vi "grSim Robot Command.vi"(9 "Array In":u8[](array[numeric]), 11 "Robots":T1) -> (1 "Array":u8[](array[numeric]))   [LabVIEW 2018]
uses:
  Convert AI Robot to Robot Command Folder/grSim/grSim Robot Command.ctl
  Varint Encoder uint32.vi
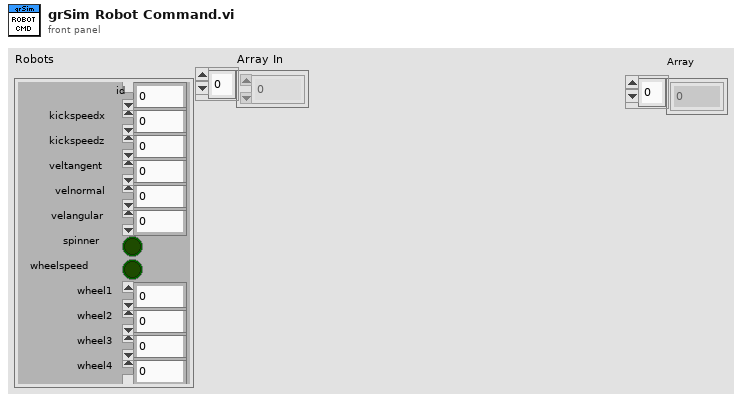
[diagram p1: front panel]
types:
  T1 = typedef "grSim Robot Command.ctl" = cluster{"id":u32, "kickspeedx":sgl, "kickspeedz":sgl, "veltangent":sgl, "velnormal":sgl, "velangular":sgl, "spinner":bool, "wheelspeed":bool, "wheel1":sgl, "wheel2":sgl, "wheel3":sgl, "wheel4":sgl}
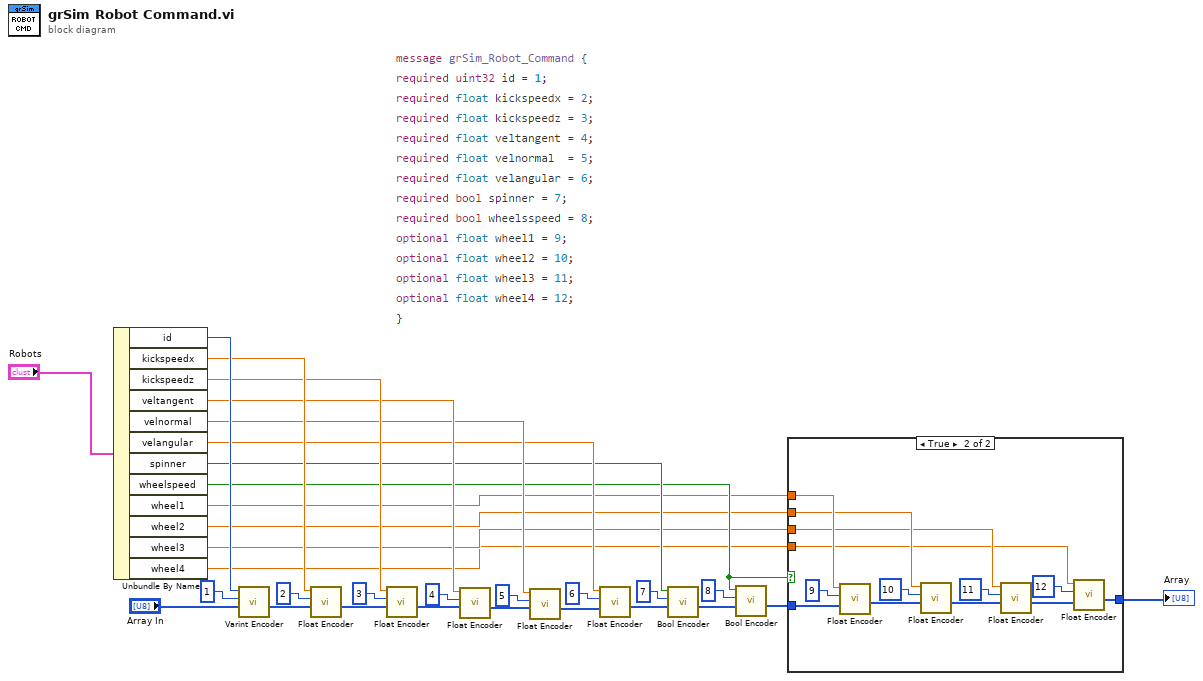
[diagram p0: block diagram]
diagram:
  n1 = Unbundle By Name("Robots") -> ("id"=w30:u32, "kickspeedx"=w25:sgl, "kickspeedz"=w16:sgl, "veltangent"=w15:sgl, "velnormal"=w14:sgl, "velangular"=w13:sgl, "spinner"=w8:bool, "wheelspeed"=w7:bool, "wheel1"=w5:sgl, "wheel2"=w4:sgl, "wheel3"=w3:sgl, "wheel4"=w2:sgl)
  n2 = call-poly "Varint Encoder.vi"("Array In"="Array In", "Key"=u32 1, "Value"=w30) -> ("Array"=w27:u8[])  [unwired: 8 in]
  n3 = call "Float Encoder.vi"("Array In"=w27, "Key"=u32 2, "Value"=w25) -> ("Array"=w20:u8[])  [unwired: 8 in]
  n4 = call "Float Encoder.vi"("Array In"=w20, "Key"=u32 3, "Value"=w16) -> ("Array"=w19:u8[])  [unwired: 8 in]
  n5 = call "Float Encoder.vi"("Array In"=w19, "Key"=u32 4, "Value"=w15) -> ("Array"=w18:u8[])  [unwired: 8 in]
  n6 = call "Float Encoder.vi"("Array In"=w18, "Key"=u32 5, "Value"=w14) -> ("Array"=w17:u8[])  [unwired: 8 in]
  n7 = call "Float Encoder.vi"("Array In"=w17, "Key"=u32 6, "Value"=w13) -> ("Array"=w12:u8[])  [unwired: 8 in]
  n8 = call "Bool Encoder.vi"("Array In"=w12, "Key"=u32 7, "Value"=w8) -> ("Array"=w10:u8[])  [unwired: 8 in]
  n9 = call "Bool Encoder.vi"("Array In"=w10, "Key"=u32 8, "Value"=w7) -> ("Array"=w6:u8[])  [unwired: 8 in]
  n10 = case shown="True" w7 {
    tunnel: w6 -> [w32 w44]
    tunnel: w5 -> [_ w37]
    tunnel: w4 -> [_ w36]
    tunnel: w3 -> [_ w35]
    tunnel: w2 -> [_ w34]
    tunnel: [w32 w33] -> w1
    frame False {
    }
    frame True {
      n11 = call "Float Encoder.vi"("Array In"=w44, "Key"=u32 9, "Value"=w37) -> ("Array"=w40:u8[])  [unwired: 8 in]
      n12 = call "Float Encoder.vi"("Array In"=w40, "Key"=u32 10, "Value"=w36) -> ("Array"=w39:u8[])  [unwired: 8 in]
      n13 = call "Float Encoder.vi"("Array In"=w39, "Key"=u32 11, "Value"=w35) -> ("Array"=w38:u8[])  [unwired: 8 in]
      n14 = call "Float Encoder.vi"("Array In"=w38, "Key"=u32 12, "Value"=w34) -> ("Array"=w33:u8[])  [unwired: 8 in]
    }
  }
  "Array" <- w1
